vi "8-Axis Roadshow Demo.vi"() -> ()   [LabVIEW 2015]
uses:
  Typedef/Typedef_Motor_Message.ctl
  EMC API/EMC_Typedef_Motor_Parameters.ctl
  Functional_Global/Typedef_Message_Queue_Action.ctl
  Functional_Global/Typedef_FPGA_Interface_Action.ctl
  Globals/Global Stop.vi
  Globals/Default Motor Parameters.vi
  <vilib>/Motion/Express/_s/nimc.ex.power.power.axis.vi
  <vilib>/Motion/Express/_s/nimc.ex.resetPosition.resetPosition.axis.vi
  <vilib>/Motion/Express/_s/nimc.ex.read.readTrajectoryData.axis.vi
  <vilib>/Motion/BlockNode/FB.NIMotion.xnode
  support/Message Queue/Message Queue.lvlib
panel:
  in  "# whole revs":dbl=3.0 format="%#_13g"
  in  "Auto Cycle Time (s)":dbl=10.0 format="%#_13g"
  in  "Auto":bool=TRUE
  in  "Mode":enum16{"Pause", "Seq 1", "Seq 2", "Seq 3"}(ring)
  in  "cts per rev":dbl=1600.0 format="%#_13g"
  in  "Stop all motors":bool
  in  "Max delay (ms)":u32=1000
  in  "Motion Parameters (Min)":T1={"position"=-10000.0, "velocity"=-10000.0, "acceleration"=50000.0, "deceleration"=50000.0, "accel. jerk"=800000.0, "decel. jerk"=800000.0}
  in  "Motion Parameters (Max)":T1={"position"=10000.0, "velocity"=10000.0, "acceleration"=100000.0, "deceleration"=100000.0, "accel. jerk"=1000000.0, "decel. jerk"=1000000.0}
  in  "Command Array":string[](array[string])=["ABS Pos Move", "REL Pos Move", "Velocity Move"]
  out "Command":T2={"Axis"="", "Motion Parameters"={"position"=1000.0, "velocity"=1000.0, "acceleration"=10000.0, "deceleration"=10000.0, "accel. jerk"=10000.0, "decel. jerk"=10000.0}}
  out "Message":string
  out "# elements in queue":i32
  out "error out":errorcluster
  out "Axis Positions":T3(graph)
  out "Axis Velocities":T3(graph)
  out "Array":dbl[](array[knob]) scale=0.0..200.0
  in  "stop":bool
  # "This example demonstrates how to set up an multi-axis SW architecture using SoftMotion.  You can have state machines that \"produce\" the motion commands, and the consumer will then digest them one at a time.\n\nIn this example, 3 producer loops generate random motion commands at random times (within 1000ms each iteration.) This VI is also meant as a stress test to see if the SM engine is robust enough for complex sequences of motion commands."
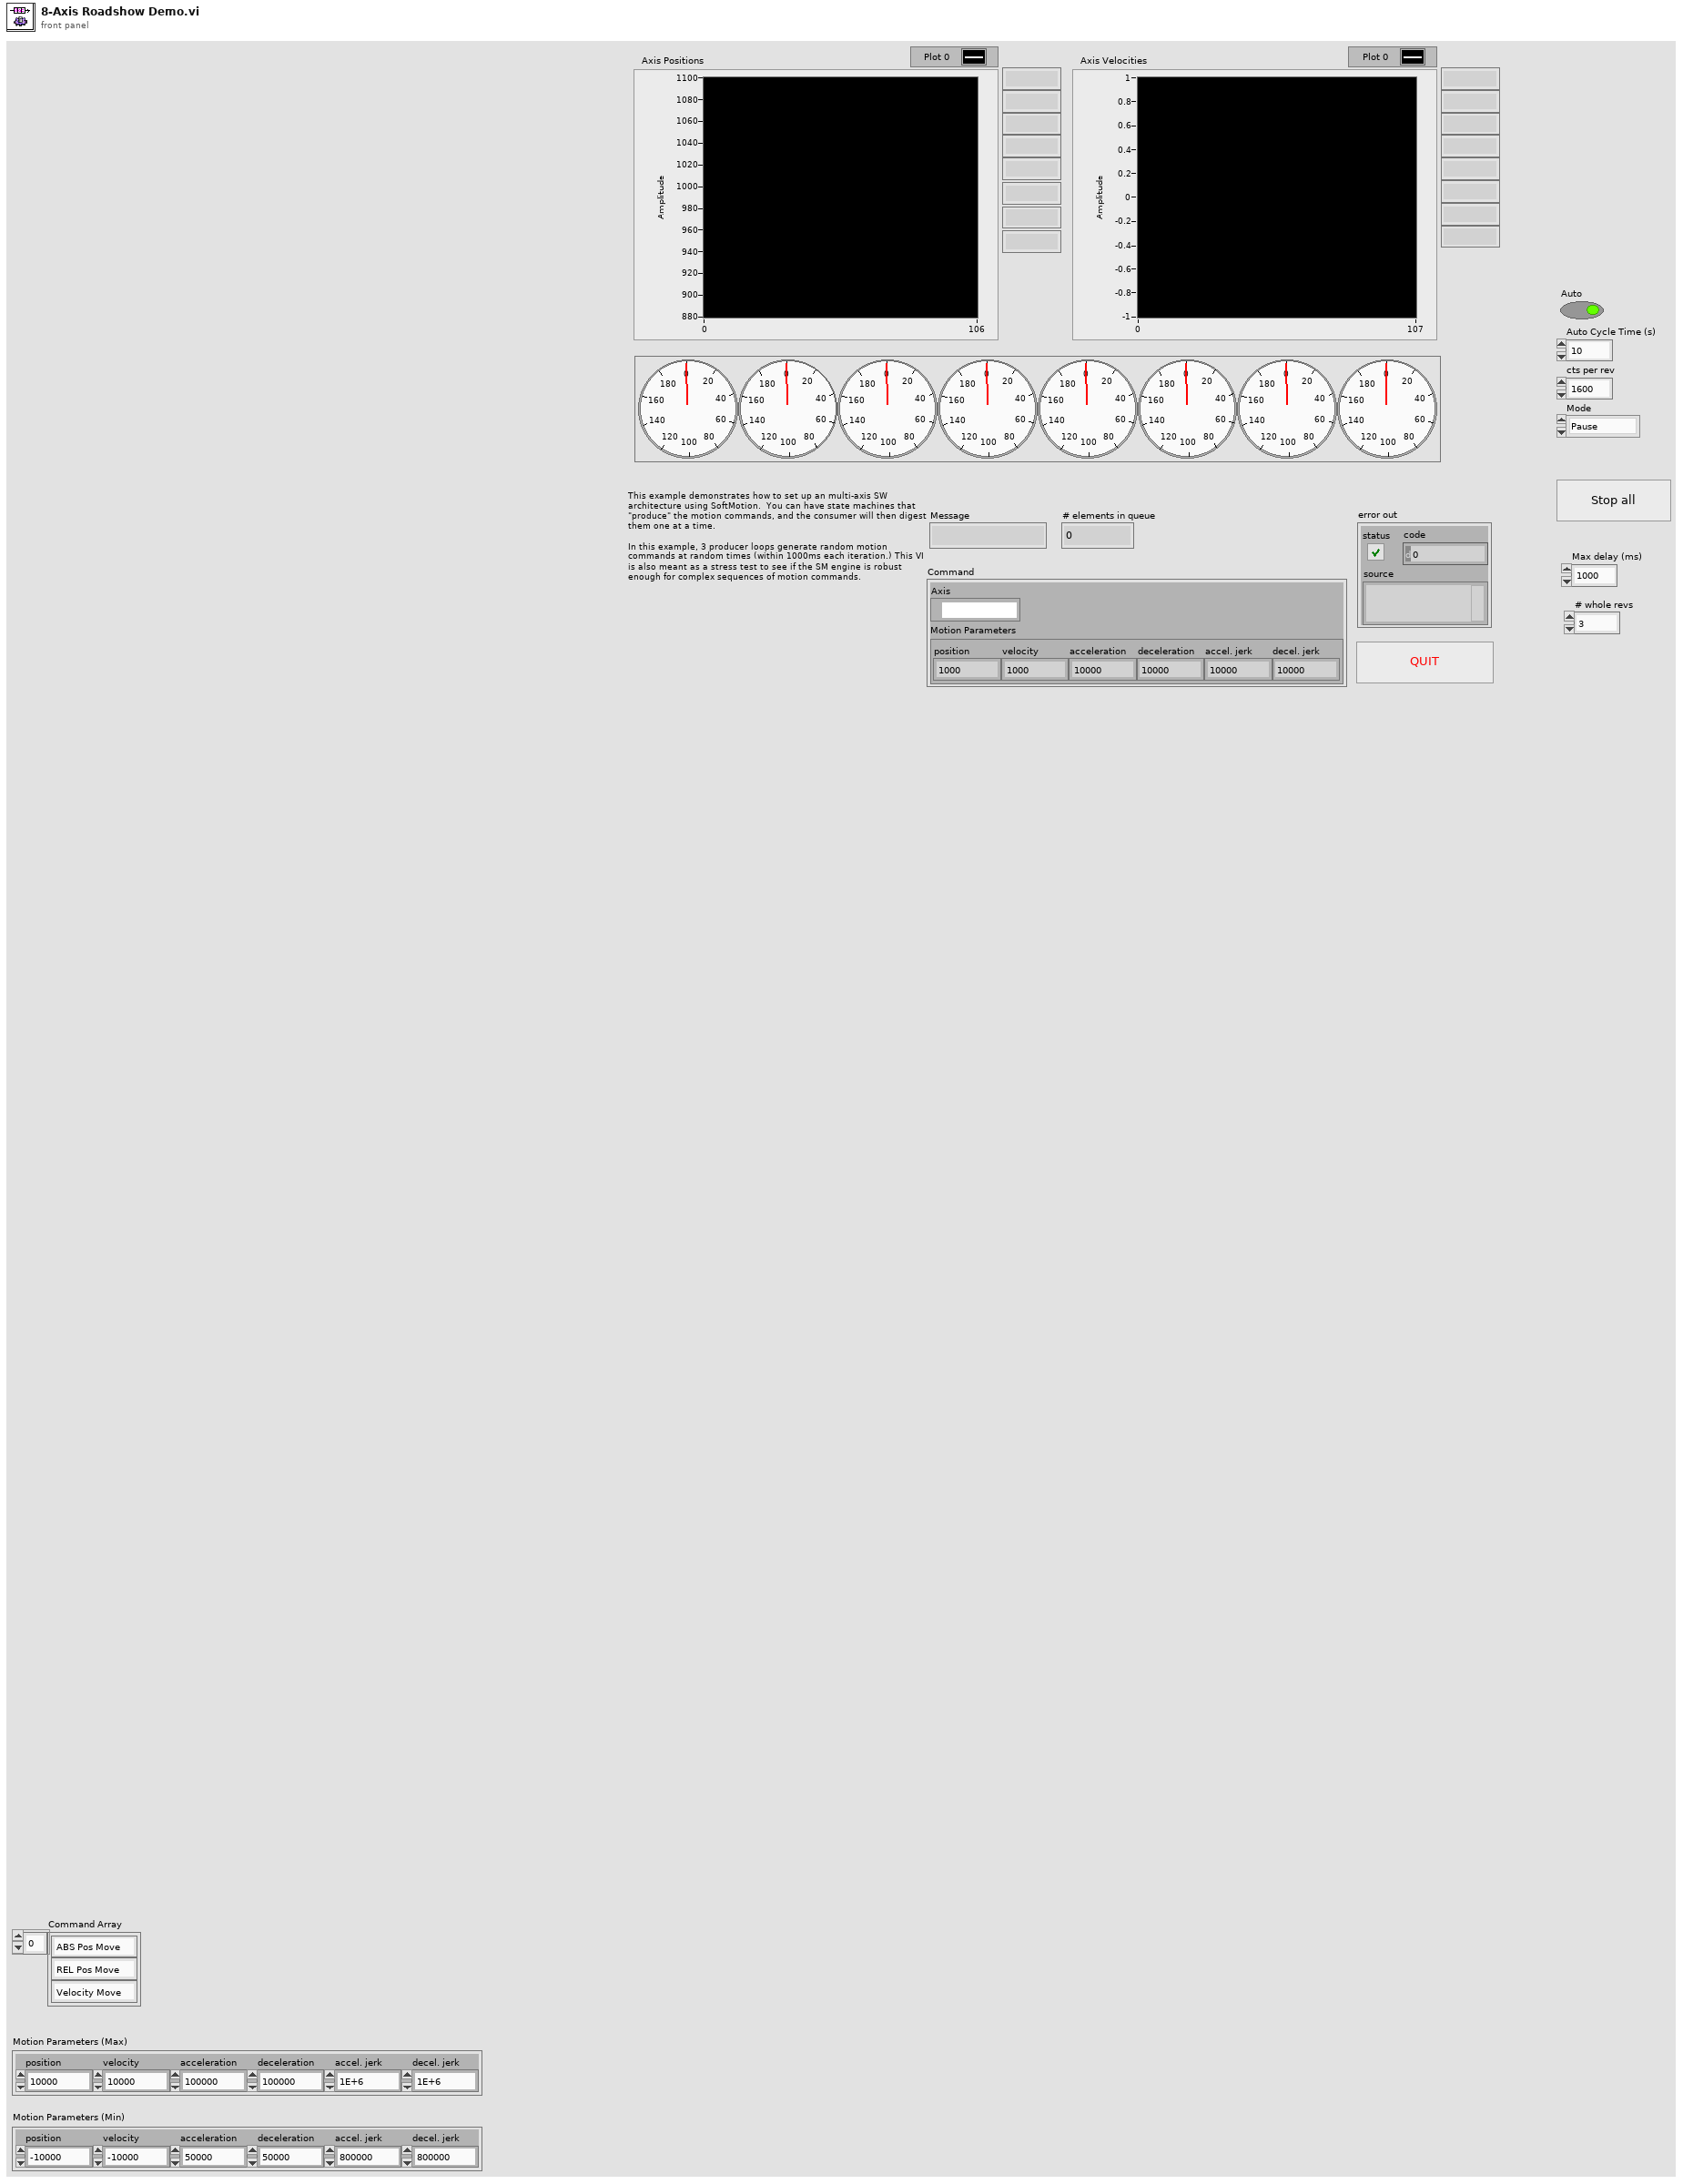
[diagram p1: front panel]
types:
  T1 = typedef "EMC_Typedef_Motor_Parameters.ctl" = cluster{"position":dbl, "velocity":dbl, "acceleration":dbl, "deceleration":dbl, "accel. jerk":dbl, "decel. jerk":dbl}
  T2 = typedef "Typedef_Motor_Message.ctl" = cluster{"Axis":refnum<k21>, "Motion Parameters":T1}
  T3 = cluster{"[0]":dbl, "[1]":dbl, "[2]":dbl, "[3]":dbl, "[4]":dbl, "[5]":dbl, "[6]":dbl, "[7]":dbl}
  T4 = typedef "Typedef_Message_Queue_Action.ctl" = enum16{"Init MQueue", "Get MQueue Ref", "Close MQueue"}
  T5 = typedef "Typedef_FPGA_Interface_Action.ctl" = enum16{"Initialize FPGA", "Get FPGA Reference", "Close FPGA"}
  T6 = typedef "Message Queue.lvlib/Message Cluster.ctl" = cluster{"Message":string, "Message Data":variant}
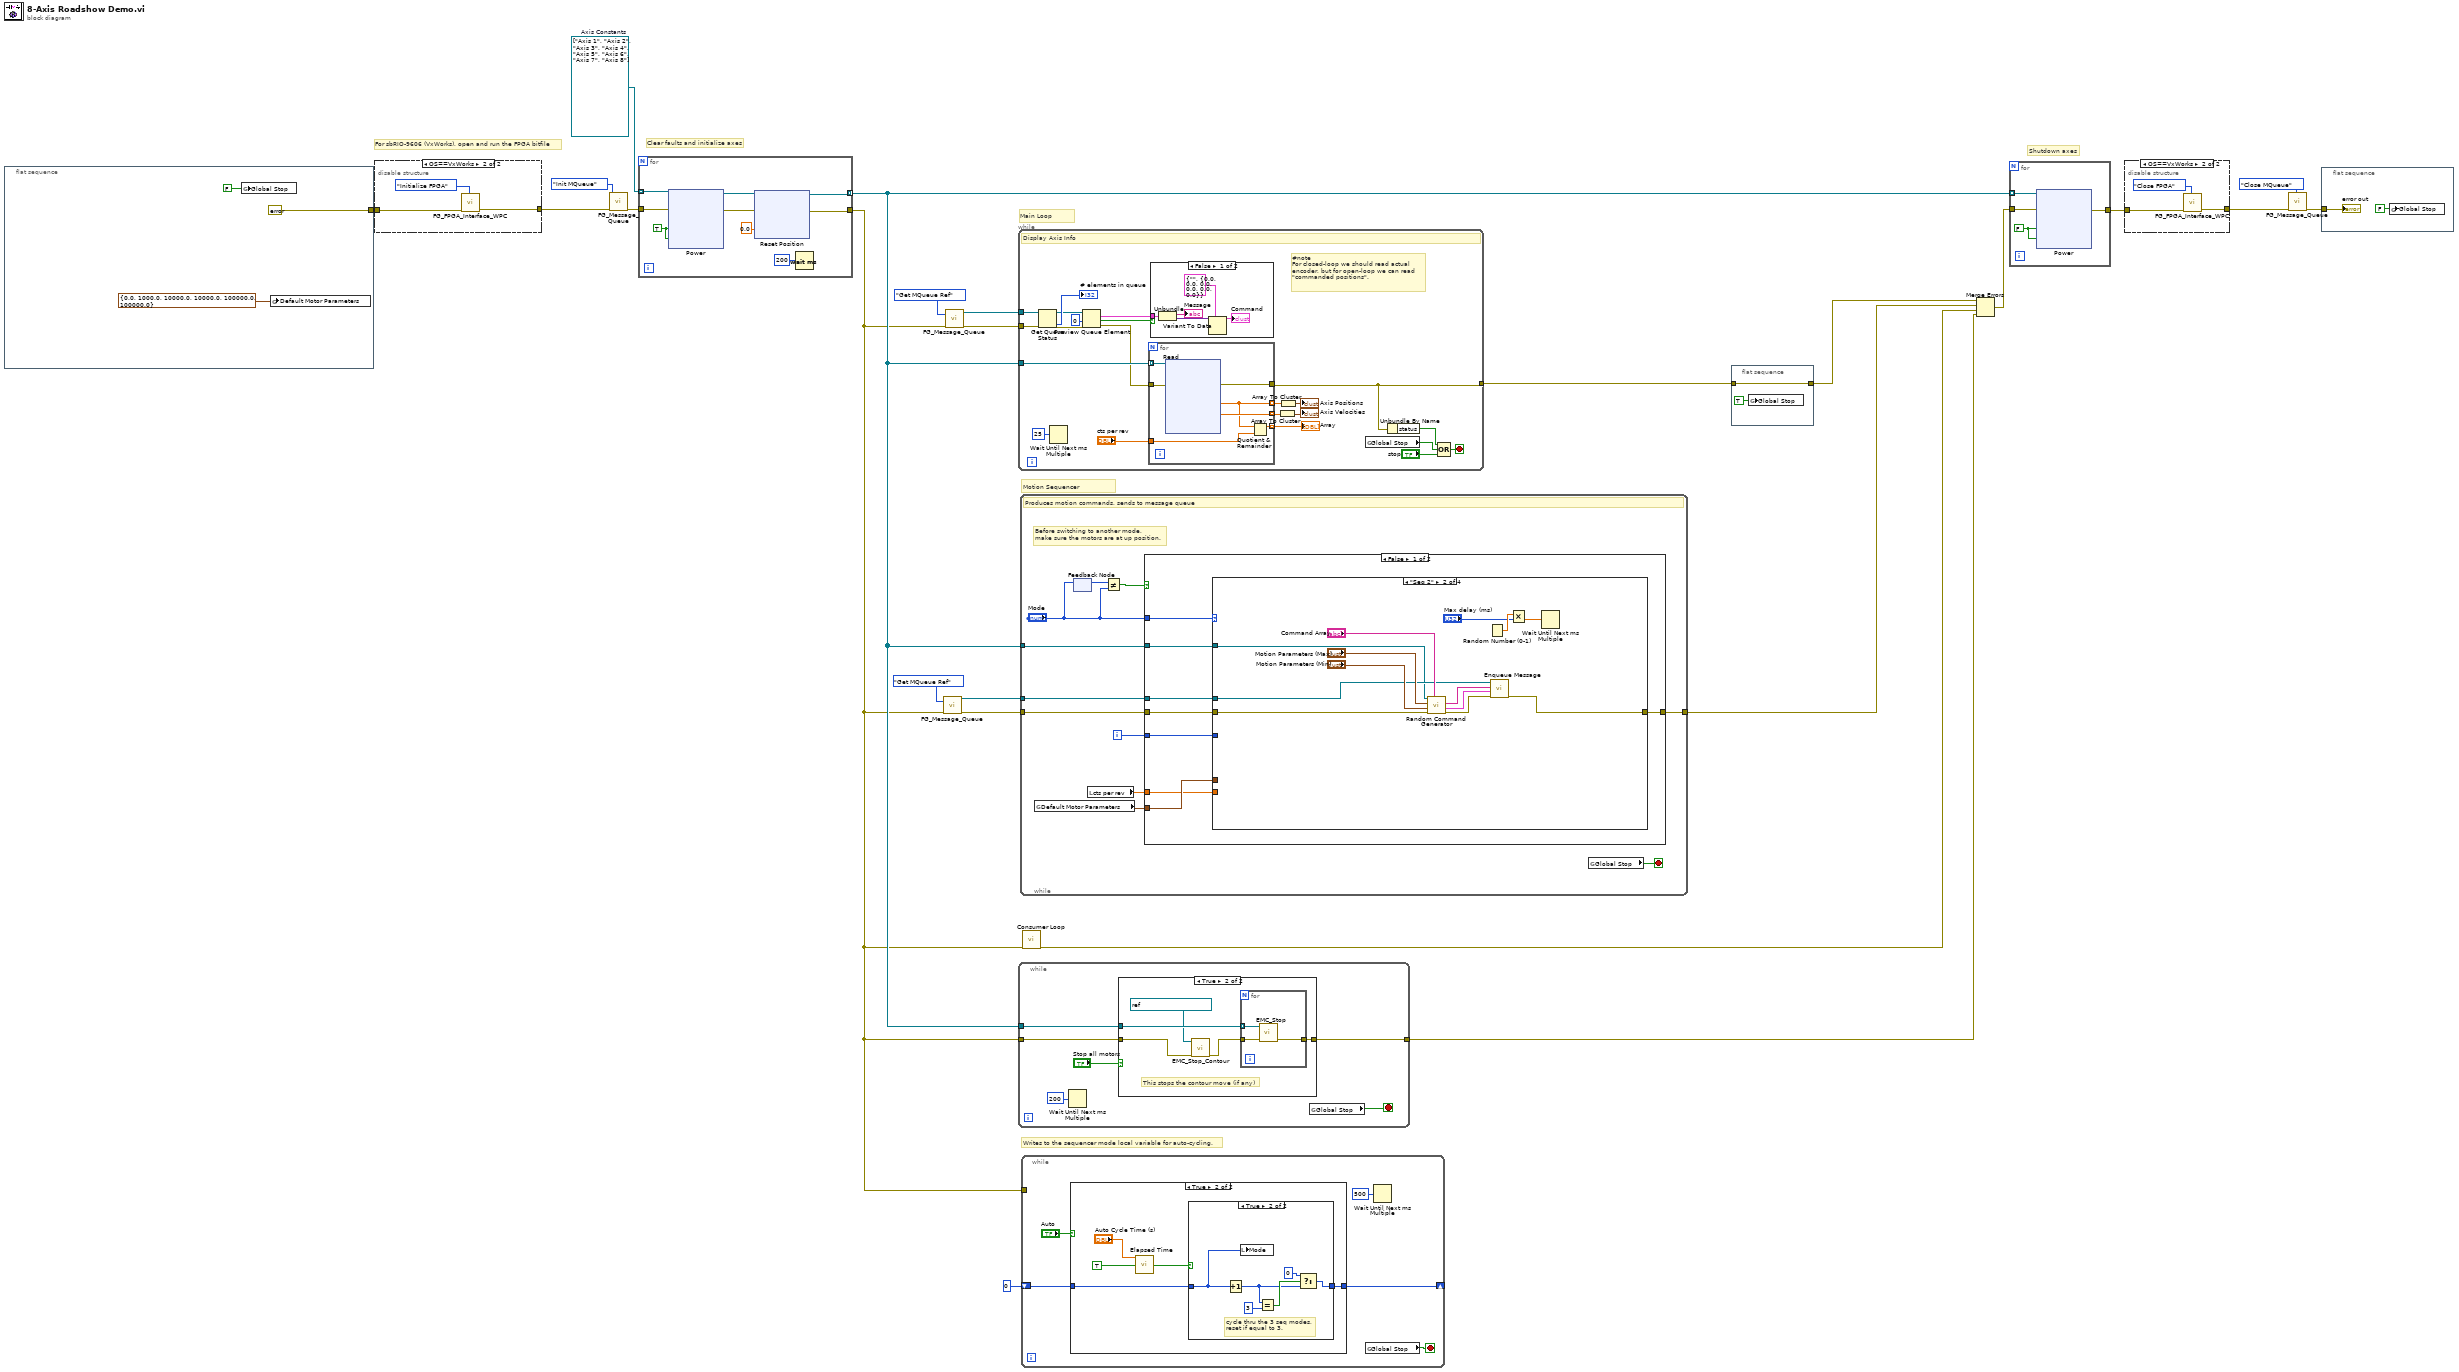
[diagram p0: block diagram]
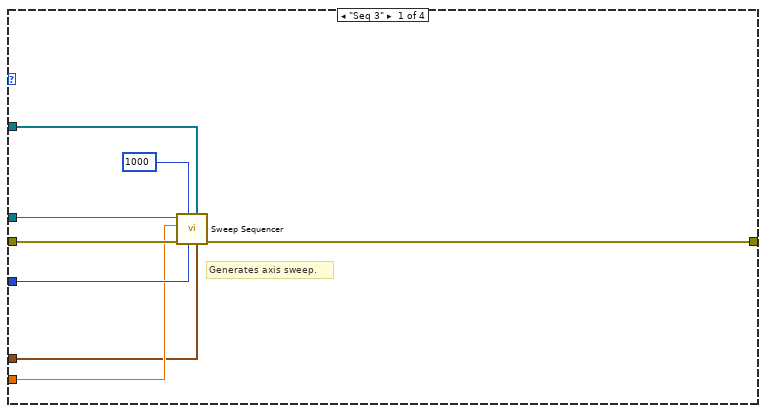
[diagram p5: hidden frame]
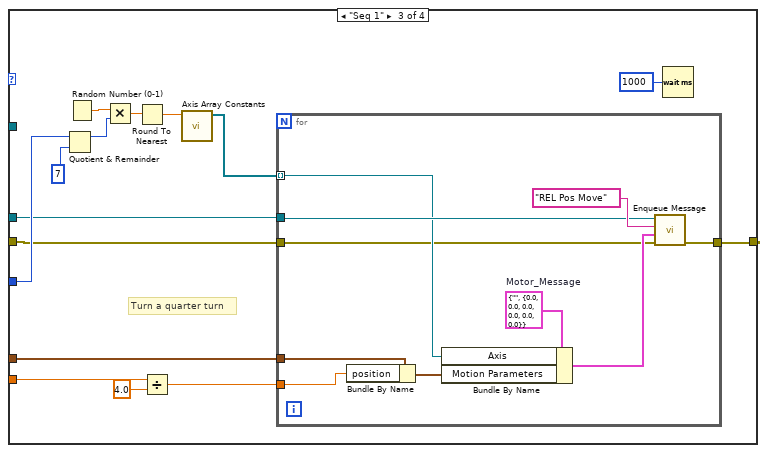
[diagram p6: hidden frame]
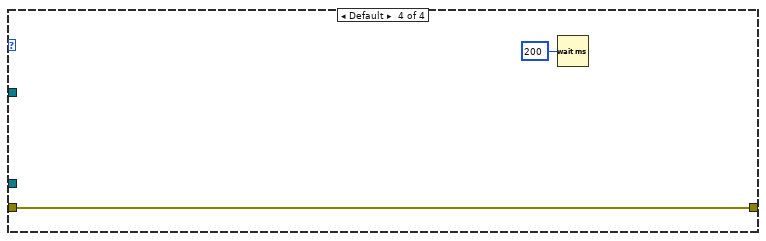
[diagram p7: hidden frame]
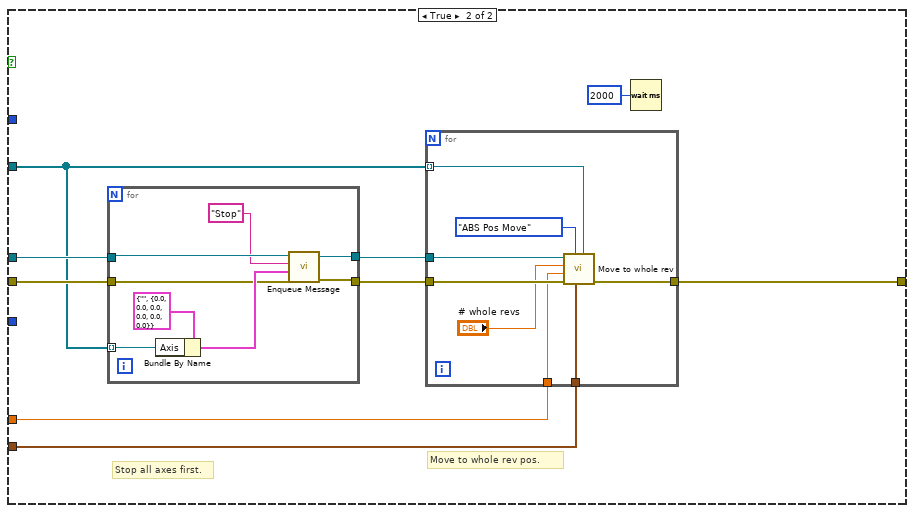
[diagram p8: hidden frame]
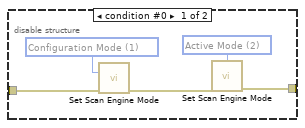
[diagram p10: hidden frame]
diagram:
  w23 = refnum<k21>[] ["Axis 1", "Axis 2", "Axis 3", "Axis 4", "Axis 5", "Axis 6", "Axis 7", "Axis 8"]  # Axis Constants
  # "Writes to the sequencer mode local variable for auto-cycling."
  # "Motion Sequencer"
  # "For sbRIO-9606 (VxWorks), open and run the FPGA bitfile"
  # "Shutdown axes"
  # "Main Loop"
  # "Clear faults and initialize axes"
  n1 = flat-sequence {
    tunnel: [errorcluster {"status"=FALSE, "code"=0, "source"=""} ("error in (no error)")] -> w24
    frame #0 {
      n2 = global write "Global Stop.vi" "Global Stop"(FALSE ("stop")) -> ()
      n3 = global write "Default Motor Parameters.vi" "Default Motor Parameters"(T1 {"position"=0.0, "velocity"=1000.0, "acceleration"=10000.0, "deceleration"=10000.0, "accel. jerk"=100000.0, "decel. jerk"=100000.0} ("Default Motor Parameters")) -> ()
    }
  }
  n4 = disable-structure shown="OS==VxWorks" {
    disable-tunnel: [w32 w33] -> w19
    disable-tunnel: w24 -> [w31 w34]
    frame condition #0 {
      w28 = 1 items=["Configuration Mode"=1, "Active Mode"=2] ("mode (Active Mode)")
      w29 = 2 items=["Configuration Mode"=1, "Active Mode"=2] ("mode (Active Mode)")
      n5 = call <vilib>:"Set Scan Engine Mode.vi"("mode (Active Mode)"=w28, "error in (no error)"=w31) -> ("error out"=w30:errorcluster)  [unwired: 13 in]
      n6 = call <vilib>:"Set Scan Engine Mode.vi"("mode (Active Mode)"=w29, "error in (no error)"=w30) -> ("error out"=w32:errorcluster)  [unwired: 13 in]
    }
    frame condition #1 (active) {
      n7 = call "FG_FPGA_Interface_WPC.vi"("Action"=Typedef_FPGA_Interface_Action."Initialize FPGA", "error in"=w34) -> ("error out"=w33:errorcluster)  [unwired: 8 in, 1 out]
    }
  }
  n8 = call "FG_Message_Queue.vi"("Action"=Typedef_Message_Queue_Action."Init MQueue", "error in"=w19) -> ("error out"=w18:errorcluster)  [unwired: 8 in, 1 out]
  n9 = for {
    tunnel: [w41] -> w2
    tunnel: [w39] -> w4 mode=indexing
    tunnel: w18 -> [w37]
    tunnel: w23 -> [w38] mode=indexing
    w44 = TRUE ("enable axis")
    n10 = xnode ("Power")("enable axis"=w44, "enable drive"=w44, "resource"=w38, "error in"=w37) -> ("resource out"=w40:refnum<k21>, "error out"=w42:errorcluster)
    n11 = xnode ("Reset Position")("position"=0.0, "resource"=w40, "error in"=w42) -> ("resource out"=w39:refnum<k21>, "error out"=w41:errorcluster)
    n12 = Wait (ms)(milliseconds to wait=u32 200) -> ()  [unwired: 1 out]
  }
  n13 = call "FG_Message_Queue.vi"("Action"=Typedef_Message_Queue_Action."Get MQueue Ref", "error in"=w2) -> ("error out"=w7:errorcluster, "Message Queue"=w6:refnum<queue>)  [unwired: 8 in]
  n14 = call "FG_Message_Queue.vi"("Action"=Typedef_Message_Queue_Action."Get MQueue Ref", "error in"=w2) -> ("error out"=w10:errorcluster, "Message Queue"=w11:refnum<queue>)  [unwired: 8 in]
  n15 = while {
    tunnel: w10 -> [w68]
    tunnel: w4 -> [w78]
    tunnel: [w62] -> w21
    tunnel: w11 -> [w70]
    stop <- w71 stop-if-true
    # "#note \nFor closed-loop we should read actual \nencoder, but for open-loop we can read\n\"commanded positions\"."
    # "Display Axis Info"
    n16 = Get Queue Status(queue=w70, error in (no error)=w68) -> (queue out=w64:refnum<queue>, error out=w66:errorcluster, # elements in queue=→"# elements in queue":i32)  [unwired: 1 in, 5 out]
    n17 = Wait Until Next ms Multiple(millisecond multiple=u32 25) -> ()  [unwired: 1 out]
    n18 = Preview Queue Element(queue=w64, timeout in ms (-1)=0, error in (no error)=w66) -> (element=w63:T6, timed out?=w61:bool, error out=w65:errorcluster)  [unwired: 1 out]
    n19 = for {
      tunnel: [w93] -> w62
      tunnel: [w89] -> w76 mode=indexing
      tunnel: [w92] -> w81 mode=indexing
      tunnel: w65 -> [w91]
      tunnel: w78 -> [w90] mode=indexing
      tunnel: [w88] -> w77 mode=indexing
      tunnel: "cts per rev" -> [w87]
      n20 = xnode ("Read")("resource"=w90, "error in"=w91) -> ("commanded position"=w89:dbl, "commanded vel."=w92:dbl, "error out"=w93:errorcluster)  [unwired: 2 out]
      n21 = Quotient & Remainder(x=w89, y=w87) -> (x-y*floor(x/y)=w88:dbl)  [unwired: 1 out]
    }
    "Array" <- w77
    n22 = case shown="False" w61 {
      tunnel: w63 -> [w86 _]
      frame False {
        n23 = Unbundle(w86) -> ("Message"=→"Message":string, "Message Data"=w83:variant)
        n24 = Variant To Data(type=T2 {"Axis"="", "Motion Parameters"={"position"=0.0, "velocity"=0.0, "acceleration"=0.0, "deceleration"=0.0, "accel. jerk"=0.0, "decel. jerk"=0.0}} ("Motor_Message"), Variant=w83) -> (data=→"Command":T2)  [unwired: 1 in, 1 out]
      }
      frame True {
      }
    }
    n25 = Array To Cluster(array=w81) -> (cluster=→"Axis Velocities":T3)
    n26 = Array To Cluster(array=w76) -> (cluster=→"Axis Positions":T3)
    n27 = global read "Global Stop.vi" "Global Stop"() -> (w72:bool)
    n28 = Unbundle By Name(w62) -> ("status"=w73:bool)
    n29 = Compound Arithmetic op=OR(w73, w72, "stop") -> (w71:bool)
  }
  n30 = while {
    tunnel: w2 -> [w106]
    tunnel: w4 -> [w104]
    tunnel: [w103] -> w3
    stop <- w102 stop-if-true
    n31 = Wait Until Next ms Multiple(millisecond multiple=u32 200) -> ()  [unwired: 1 out]
    n32 = case shown="True" "Stop all motors" {
      tunnel: w106 -> [w107 w110]
      tunnel: [w107 w112] -> w103
      tunnel: w104 -> [_ w111]
      frame False {
      }
      frame True {
        # "This stops the contour move (if any)"
        n33 = call "EMC_Stop_Contour.vi"("error in (no error)"=w110, "coordinate"=refnum<k21> "Coordinate Space 1") -> ("error out"=w108:errorcluster)  [unwired: 9 in]
        n34 = for {
          tunnel: w108 -> [w115]
          tunnel: w111 -> [w113] mode=indexing
          tunnel: [w114] -> w112
          n35 = call "EMC_Stop.vi"("error in (no error)"=w115, "axis"=w113) -> ("error out"=w114:errorcluster)  [unwired: 8 in, 1 out]
        }
      }
    }
    n36 = global read "Global Stop.vi" "Global Stop"() -> (w102:bool)
  }
  n37 = while {
    tunnel: w4 -> [w123]
    tunnel: w7 -> [w125]
    tunnel: w6 -> [w124]
    tunnel: [w121] -> w5
    i -> [w122]
    stop <- w126 stop-if-true
    # "Before switching to another mode,\nmake sure the motors are at up position."
    # "Produces motion commands, sends to message queue"
    n38 = global read "Default Motor Parameters.vi" "Default Motor Parameters"() -> (w118:T1)
    n39 = feedback-in #1("Mode") -> ()
    n40 = feedback #1() -> (w120:enum16{"Pause", "Seq 1", "Seq 2", "Seq 3"})  [unwired: 1 in]
    n41 = local read "cts per rev"() -> (w116:dbl)
    n42 = Not Equal?(x=w120, y="Mode") -> (x != y?=w119:bool)
    n43 = case shown="False" w119 {
      tunnel: w125 -> [w134 w188]
      tunnel: w124 -> [w133 w189]
      tunnel: w123 -> [w132 w185]
      tunnel: w122 -> [w131 _]
      tunnel: [w130 w191] -> w121
      tunnel: "Mode" -> [w129 _]
      tunnel: w118 -> [w128 w184]
      tunnel: w116 -> [w127 w183]
      frame False {
        n44 = case shown="\"Seq 2\"" w129 {
          tunnel: w134 -> [w142 w149 w168 w181]
          tunnel: w133 -> [w140 w148 w166 _]
          tunnel: w132 -> [w138 w147 _ _]
          tunnel: w131 -> [w141 _ w169 _]
          tunnel: [w139 w144 w167 w181] -> w130
          tunnel: w128 -> [w135 _ w161 _]
          tunnel: w127 -> [w136 _ w160 _]
          frame "Seq 3" {
            # "Generates axis sweep."
            n45 = call "Sweep Sequencer.vi"("Default Motor Parameters"=w135, "Axis Array"=w138, "Loop counter in"=w141, "Max delay (ms)"=u32 1000, "error in (no error)"=w142, "cts per rev"=w136, "Message Queue"=w140) -> ("error out"=w139:errorcluster)  [unwired: 4 in]
          }
          frame "Seq 2" {
            n46 = call "Random Command Generator.vi"("Command Array"="Command Array", "error in (no error)"=w149, "Motion Parameters (Min)"="Motion Parameters (Min)", "Motion Parameters (Max)"="Motion Parameters (Max)", "Axis Resources"=w147) -> ("error out"=w150:errorcluster, "Motor_Message"=w152:T2, "Command Out"=w151:string)  [unwired: 4 in]
            n47 = Random Number (0-1)() -> (number: 0 to 1=w145:dbl)
            n48 = call "Enqueue Message.vi"("error in (no error)"=w150, "Message Data"=w152, "Message"=w151, "Message Queue"=w148) -> ("error out"=w144:errorcluster)  [unwired: 6 in, 1 out]
            n49 = Multiply(x=w145, y="Max delay (ms)") -> (x*y=w146:dbl)
            n50 = Wait Until Next ms Multiple(millisecond multiple=w146) -> ()  [unwired: 1 out]
          }
          frame "Seq 1" {
            # "Turn a quarter turn"
            n51 = Quotient & Remainder(x=w169, y=7) -> (x-y*floor(x/y)=w163:i32)  [unwired: 1 out]
            n52 = Random Number (0-1)() -> (number: 0 to 1=w164:dbl)
            n53 = Multiply(x=w164, y=w163) -> (x*y=w162:dbl)
            n54 = Round To Nearest(number=w162) -> (nearest integer value=w156:dbl)
            n55 = Divide(x=w160, y=4.0) -> (x/y=w158:dbl)
            n56 = call "Axis Array Constants.vi"("Numeric"=w156) -> ("Axis Constants"=w157:refnum<k21>[])  [unwired: 10 in]
            n57 = for {
              tunnel: w157 -> [w175] mode=indexing
              tunnel: w168 -> [w174]
              tunnel: [w173] -> w167
              tunnel: w158 -> [w176]
              tunnel: w166 -> [w177]
              tunnel: w161 -> [w171]
              w180 = T2 {"Axis"="", "Motion Parameters"={"position"=0.0, "velocity"=0.0, "acceleration"=0.0, "deceleration"=0.0, "accel. jerk"=0.0, "decel. jerk"=0.0}}  # Motor_Message
              n58 = Bundle By Name(cluster=w171, "position"=w176) -> (w172:T1)
              n59 = Bundle By Name(cluster=w180, "Axis"=w175, "Motion Parameters"=w172) -> (w179:T2)
              n60 = call "Enqueue Message.vi"("error in (no error)"=w174, "Message Data"=w179, "Message"="REL Pos Move", "Message Queue"=w177) -> ("error out"=w173:errorcluster)  [unwired: 6 in, 1 out]
            }
            n61 = Wait (ms)(milliseconds to wait=u32 1000) -> ()  [unwired: 1 out]
          }
          frame Default {
            n62 = Wait (ms)(milliseconds to wait=u32 200) -> ()  [unwired: 1 out]
          }
        }
      }
      frame True {
        # "Move to whole rev pos."
        # "Stop all axes first."
        n63 = for {
          tunnel: w189 -> [w199]
          tunnel: w188 -> [w193]
          tunnel: [w192] -> w187
          tunnel: [w197] -> w186
          tunnel: w185 -> [w194] mode=indexing
          n64 = Bundle By Name(cluster=T2 {"Axis"="", "Motion Parameters"={"position"=0.0, "velocity"=0.0, "acceleration"=0.0, "deceleration"=0.0, "accel. jerk"=0.0, "decel. jerk"=0.0}} ("Motor_Message"), "Axis"=w194) -> (w195:T2)
          n65 = call "Enqueue Message.vi"("error in (no error)"=w193, "Message Data"=w195, "Message"="Stop", "Message Queue"=w199) -> ("error out"=w192:errorcluster, "dup Message Queue"=w197:refnum<queue>)  [unwired: 6 in]
        }
        n66 = for {
          tunnel: w185 -> [w203] mode=indexing
          tunnel: w187 -> [w207]
          tunnel: [w206] -> w191
          tunnel: w186 -> [w205]
          tunnel: w184 -> [w202]
          tunnel: w183 -> [w201]
          n67 = call "Move to whole rev.vi"("resource in"=w203, "Default Motor Parameters"=w202, "Mode"=enum16{"ABS Pos Move", "REL Pos Move"}."ABS Pos Move", "error in (no error)"=w207, "cts per rev"=w201, "# whole revs"="# whole revs", "Queue in"=w205) -> ("error out"=w206:errorcluster)  [unwired: 3 in, 1 out]
        }
        n68 = Wait (ms)(milliseconds to wait=u32 2000) -> ()  [unwired: 1 out]
      }
    }
    n69 = global read "Global Stop.vi" "Global Stop"() -> (w126:bool)
  }
  n70 = while {
    tunnel: w2 -> [_]
    shift-right: [w209] -> _
    shift-left: 0 -> [w210]
    stop <- w212 stop-if-true
    n71 = case shown="True" "Auto" {
      tunnel: w210 -> [w213 w216]
      tunnel: [w213 w215] -> w209
      frame False {
      }
      frame True {
        n72 = call "Elapsed Time"("Time Target (s)"="Auto Cycle Time (s)", "Auto Reset"=TRUE) -> ("Time has Elapsed"=w217:bool)  [unwired: 10 in, 7 out]
        n73 = case shown="True" w217 {
          tunnel: w216 -> [w219 w225]
          tunnel: [w219 w220] -> w215
          frame False {
          }
          frame True {
            # "cycle thru the 3 seq modes,\nreset if equal to 3."
            n74 = Increment(x=w225) -> (x+1=w222:i32)
            n75 = local write "Mode"(w225) -> ()
            n76 = Equal?(x=w222, y=3) -> (x = y?=w223:bool)
            n77 = Select(t=0, s=w223, f=w222) -> (s? t:f=w220:i32)
          }
        }
      }
    }
    n78 = global read "Global Stop.vi" "Global Stop"() -> (w212:bool)
    n79 = Wait Until Next ms Multiple(millisecond multiple=u32 500) -> ()  [unwired: 1 out]
  }
  n80 = call "Consumer Loop.vi"("error in (no error)"=w2) -> ("error out"=w9:errorcluster)  [unwired: 10 in]
  n81 = flat-sequence {
    tunnel: w21 -> [w226]
    tunnel: [w226] -> w13
    frame #0 {
      n82 = global write "Global Stop.vi" "Global Stop"(TRUE ("stop")) -> ()
    }
  }
  n83 = Merge Errors(w13, w5, w9, w3) -> (w17:errorcluster)
  n84 = for {
    tunnel: w4 -> [w231] mode=indexing
    tunnel: [w229] -> w22
    tunnel: w17 -> [w228]
    w230 = FALSE ("enable axis")
    n85 = xnode ("Power")("enable axis"=w230, "enable drive"=w230, "resource"=w231, "error in"=w228) -> ("error out"=w229:errorcluster)  [unwired: 1 out]
  }
  n86 = disable-structure shown="OS==VxWorks" {
    disable-tunnel: [w242 w243] -> w15
    disable-tunnel: w22 -> [w242 w244]
    frame condition #0 {
    }
    frame condition #1 (active) {
      n87 = call "FG_FPGA_Interface_WPC.vi"("Action"=Typedef_FPGA_Interface_Action."Close FPGA", "error in"=w244) -> ("error out"=w243:errorcluster)  [unwired: 8 in, 1 out]
    }
  }
  n88 = call "FG_Message_Queue.vi"("Action"=Typedef_Message_Queue_Action."Close MQueue", "error in"=w15) -> ("error out"=w14:errorcluster)  [unwired: 8 in, 1 out]
  n89 = flat-sequence {
    tunnel: w14 -> [w246]
    frame #0 {
      n90 = global write "Global Stop.vi" "Global Stop"(FALSE ("stop")) -> ()
      "error out" <- w246
    }
  }
